vi "CorrFactor.vi"() -> ()   [LabVIEW 2018, in "Visualization.lvlib" / "VisualizeAnalysis.lvclass"]
uses:
  VisualizeAnalysis.lvclass
  VisualizeBase/VisualizeBase_class/SubVIs/VisualizationOptions.ctl
  <vilib>/Utility/miscctls.llb/LVRectTypeDef.ctl
  VisualizeBase/VisualizeBase_class/Requests/VisUserEventType.ctl
  <vilib>/event_ctls.llb/usereventprio.ctl
  <extravilib>/ChannelInstances/Tag-bool/Write With Abort.vi
  <extravilib>/ChannelInstances/Tag-bool/Read With Abort.vi
  <extravilib>/ChannelInstances/Tag-bool/Instantiate.vi
  <extravilib>/ChannelInstances/Tag-bool/EndpointRead.vi
  <vilib>/Utility/error.llb/Error Cluster From Error Code.vi
  <extravilib>/ChannelInstances/Tag-bool/Endpoint.vi
  <vilib>/ErrorRing/Error Ring.xnode
  VisualizeBase/VisualizeBase_class/VisualizeBase.lvclass
  Analysis/AnalysisModule/AnalysisModule.lvlib
  <userlib>/NIST/NISTErrorLib/NISTErrorLib.lvlib
  StatusAndLog/VisualizeStatus.lvclass
  <extravilib>/ChannelInstances/Tag-bool.lvlib
panel:
  in  "Log Data":bool=TRUE
  in  "btnReset":bool
  out "ROCOF":cluster{"Freq":dbl, "Freq":dbl}[](graph)
  out "Freq":cluster{"Freq":dbl, "Freq":dbl}[](graph)
  in  "PluginName":string="Sensor.RoomAlert1"
  in  "btnClearTest":bool
  in  "btnPause":bool
  in  "btnOpen":bool
  in  "INIFilePath":path
  out "VisualizationProperties":T1={"PauseAtStartup"=TRUE, "LogData"=FALSE, "LaunchInSubPanel"=TRUE, "FPMonitor"=0, "FPWindowBounds"={"Left"=0, "Top"=0, "Right"=0, "Bottom"=0}, "MonitorBounds"={"Left"=0, "Top"=0, "Right"=0, "Bottom"=0}}
  in  "ModuleID":i32
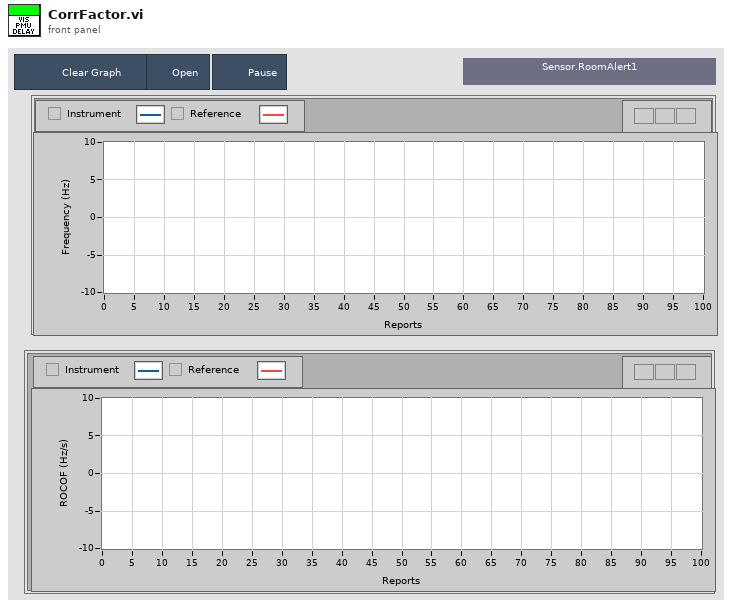
[diagram p1: front panel]
types:
  T1 = typedef "Visualization.lvlib/VisualizeBase.lvclass/VisualizationOptions.ctl" = cluster{"PauseAtStartup":bool, "LogData":bool, "LaunchInSubPanel":bool, "FPMonitor":u16, "FPWindowBounds":T2, "MonitorBounds":cluster{"Left":i16, "Top":i16, "Right":i16, "Bottom":i16}}
  T2 = typedef "LVRectTypeDef.ctl" = cluster{"Left":i16, "Top":i16, "Right":i16, "Bottom":i16}
  T3 = typedef "Visualization.lvlib/VisualizeBase.lvclass/VisRequestEvents.ctl" = cluster{"StopRequest":refnum<user-event>, "ResetRequest":refnum<user-event>, "FP Pop In or Out":refnum<user-event>}
  T4 = typedef "AnalysisModule.lvlib/clBroadcastEvents.ctl" = cluster{"DidInit":refnum<user-event>, "StatusUpdate":refnum<user-event>, "ErrorReport":refnum<user-event>, "DidStop":refnum<user-event>, "PathToINI":refnum<user-event>, "Config":refnum<user-event>, "ResultReport":refnum<user-event>, "FunctionClass":refnum<user-event>, "State":refnum<user-event>, "FunctionParams":refnum<user-event>, "Duration":refnum<user-event>}
  T5 = typedef "usereventprio.ctl" = enum32{"high priority", "normal priority"}
  T6 = typedef "Visualization.lvlib/VisualizeBase.lvclass/VisUserEventType.ctl" = cluster{"BusIndex":i8, "Data":variant}
  T7 = typedef "Tag-bool.lvlib/))Channel.ctl" = refnum<queue>
  T8 = typedef "sizeaction.ctl" = enum32{"Minimized", "Maximized", "Resized"}
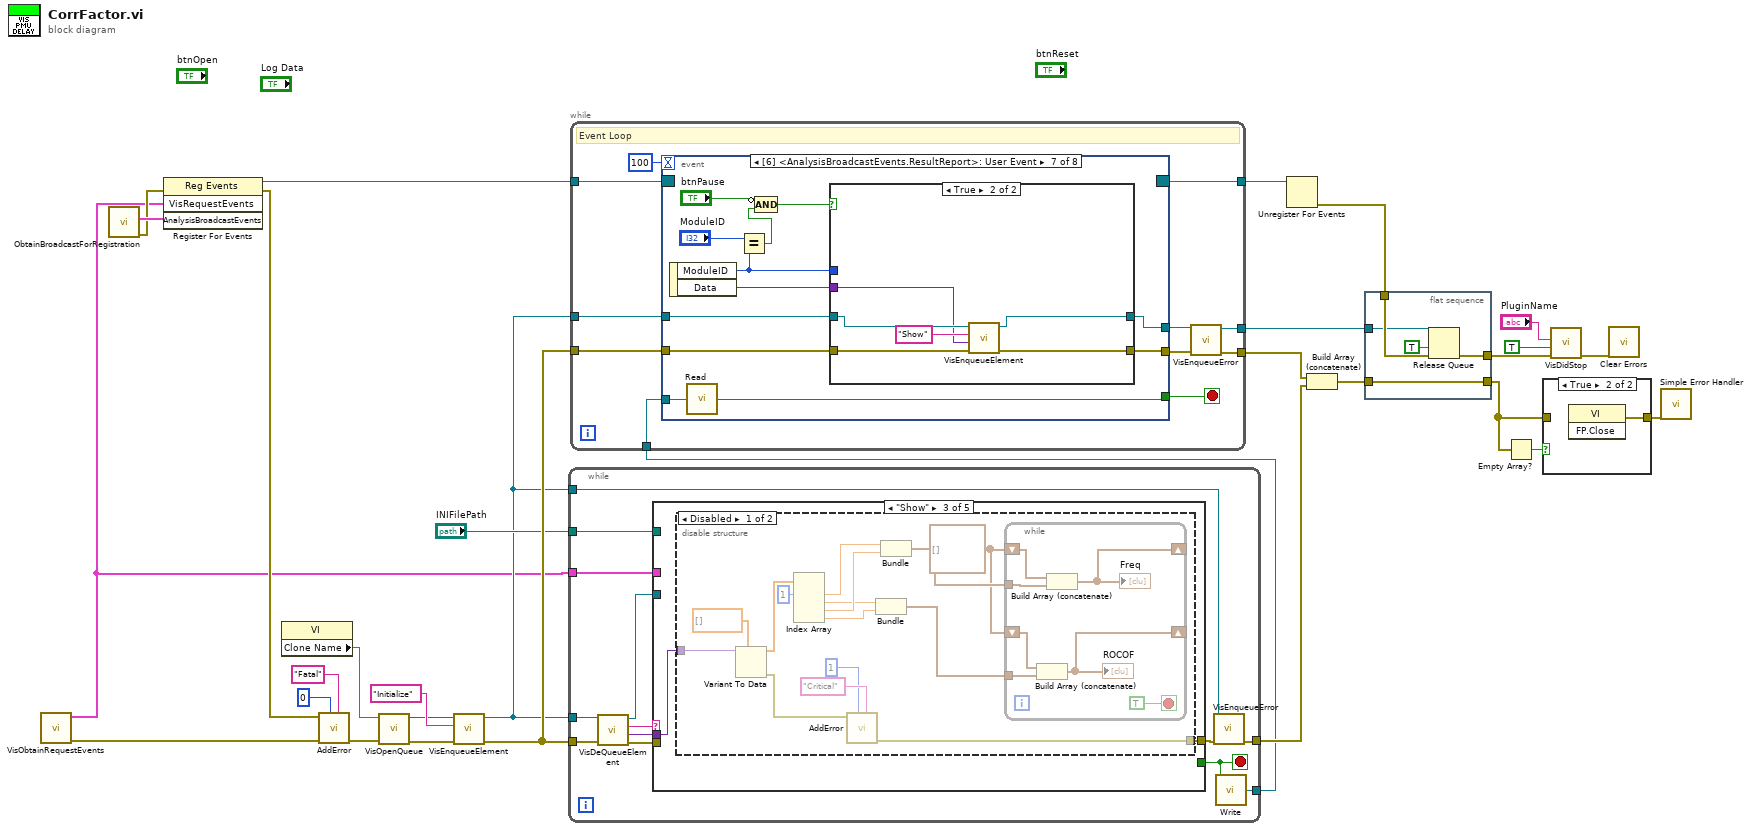
[diagram p0: block diagram]
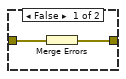
[diagram p2: hidden frame]
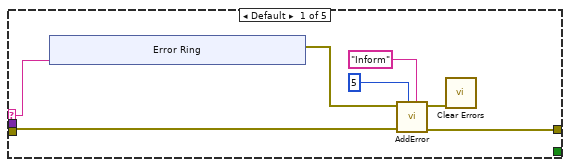
[diagram p3: hidden frame]
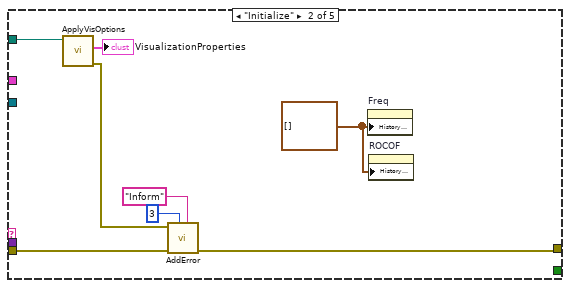
[diagram p4: hidden frame]
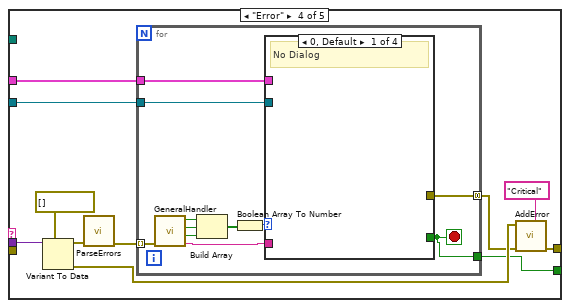
[diagram p6: hidden frame]
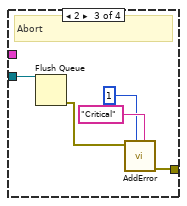
[diagram p8: hidden frame]
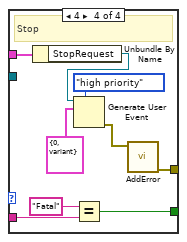
[diagram p9: hidden frame]
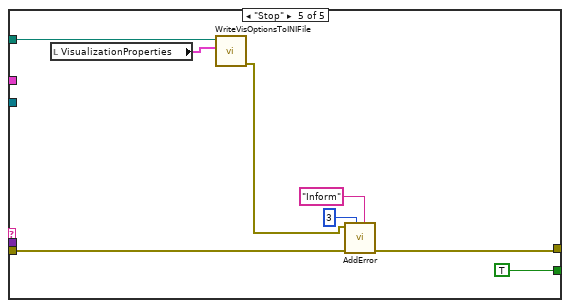
[diagram p10: hidden frame]
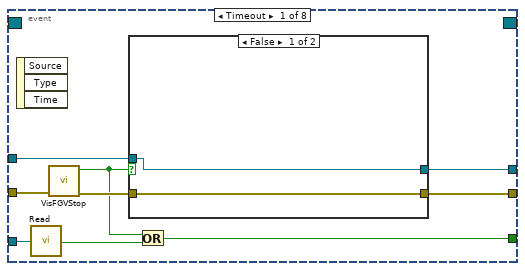
[diagram p11: hidden frame]
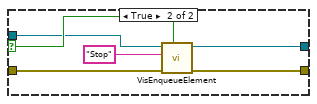
[diagram p12: hidden frame]
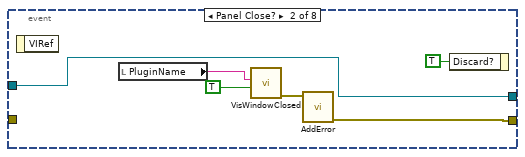
[diagram p13: hidden frame]
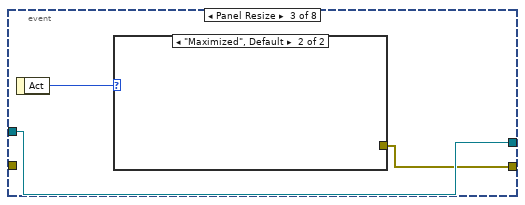
[diagram p14: hidden frame]
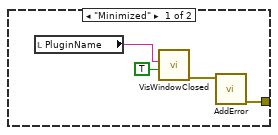
[diagram p15: hidden frame]
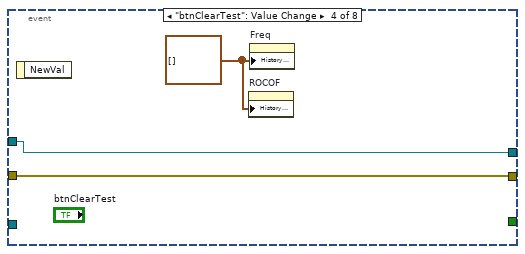
[diagram p16: hidden frame]
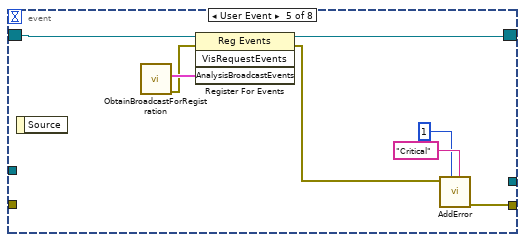
[diagram p17: hidden frame]
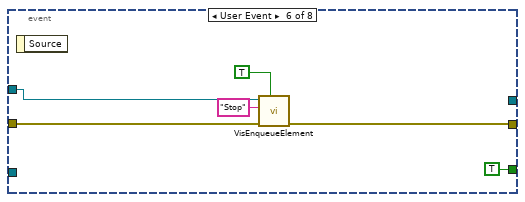
[diagram p18: hidden frame]
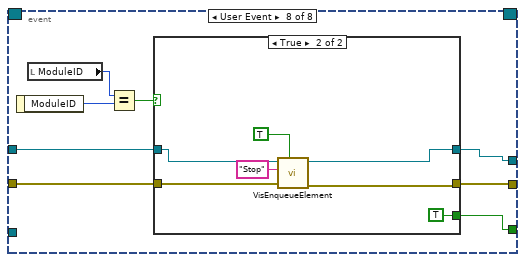
[diagram p20: hidden frame]
diagram:
  n1 = call "VisObtainRequestEvents.vi"() -> ("Error"=w29:errorcluster[], "VisRequestEvents"=w8:T3)  [unwired: 10 in]
  n2 = call "ObtainBroadcastForRegistration.vi"() -> ("error out"=w28:errorcluster, "AnalysisBroadcastEvents"=w30:T4)  [unwired: 10 in]
  n3 = register-events(error in=w28, w8, w30) -> (reference out=w20:refnum<event-registration>, error out=w27:errorcluster)  [unwired: 1 in]
  n4 = property class="VI"() -> ("Clone Name"=w22:string)  [unwired: 2 in, 2 out]
  n5 = call <userlib>:"AddError.vi"("Severity"="Fatal", "Priority"=u8 0, "ErrorArray In"=w29, "error in (no error)"=w27) -> ("ErrorArray Out"=w24:errorcluster[])  [unwired: 6 in, 1 out]
  n6 = call "VisOpenQueue.vi"("Error Array In"=w24, "QueueName"=w22) -> ("Error Array Out"=w23:errorcluster[], "queue out"=w19:refnum<queue>)  [unwired: 8 in]
  n7 = call "VisEnqueueElement.vi"("Error Array In"=w23, "Message"="Initialize", "queue in"=w19) -> ("Error Array Out"=w17:errorcluster[], "queue out"=w9:refnum<queue>)  [unwired: 7 in]
  n8 = while {
    tunnel: w17 -> [w43]
    tunnel: w9 -> [w42]
    tunnel: "INIFilePath" -> [w38]
    tunnel: [w34] -> w12
    tunnel: [w36] -> w10
    tunnel: w9 -> [w33]
    tunnel: w8 -> [w32]
    stop <- w37 stop-if-true
    n9 = call "VisDeQueueElement.vi"("Error Array In"=w43, "Queue In"=w42) -> ("Error Array Out"=w41:errorcluster[], "Data"=w40:variant, "Message"=w39:string, "Queue Out"=w31:refnum<queue>)  [unwired: 6 in]
    n10 = case shown="\"Show\"" w39 {
      selector: w39 -> [w44 _ _ _ _]
      tunnel: w41 -> [w46 w63 _ _ w131]
      tunnel: w40 -> [_ _ w67 w100 _]
      tunnel: w38 -> [_ w65 _ _ w133]
      tunnel: [w45 w59 w66 w95 w127] -> w35
      tunnel: [_ _ _ w92 TRUE] -> w37
      tunnel: w32 -> [_ _ _ w96 _]
      tunnel: w31 -> [_ _ _ w90 _]
      frame Default {
        n11 = xnode "Error Ring"("parameter 0"=w44) -> ("error out"=w50:errorcluster)
        n12 = call <userlib>:"AddError.vi"("Severity"="Inform" ("String"), "Priority"=u8 5, "ErrorArray In"=w46, "error in (no error)"=w50) -> ("ErrorArray Out"=w45:errorcluster[], "error out"=w49:errorcluster)  [unwired: 6 in]
        n13 = call <vilib>:"Clear Errors.vi"("error in (no error)"=w49) -> ()  [unwired: 5 in, 2 out]
      }
      frame "Initialize" {
        w58 = cluster{"Freq":dbl, "Freq":dbl}[] [] ("History Data")
        n14 = call "ApplyVisOptions.vi"("INIFilePath"=w65) -> ("error out"=w62:errorcluster, "VisualizationProperties"=→"VisualizationProperties":T1)  [unwired: 9 in]
        n15 = call <userlib>:"AddError.vi"("Severity"="Inform", "Priority"=u8 3, "ErrorArray In"=w63, "error in (no error)"=w62) -> ("ErrorArray Out"=w59:errorcluster[])  [unwired: 6 in, 1 out]
        n16 = property on="Freq" class="WFChart (strict)"("History Data"=w58) -> ()  [unwired: 2 in, 2 out]
        n17 = property on="ROCOF" class="WFChart (strict)"("History Data"=w58) -> ()  [unwired: 2 in, 2 out]
      }
      frame "Show" {
        n18 = disable-structure shown="Disabled" {
          disable-tunnel: w67 -> [w82 _]
          disable-tunnel: [w80 _] -> w66
          frame Disabled {
            w68 = cluster{"Freq":dbl, "Freq":dbl}[] []
            n19 = Variant To Data(type=dbl[] [], Variant=w82) -> (data=w76:dbl[], error out=w79:errorcluster)  [unwired: 1 in]
            n20 = Index Array(array=w76, index #1=1 ("index")) -> (element #1=w74:dbl, element #2=w72:dbl, element #3=w73:dbl, element #4=w71:dbl)  [unwired: 3 in]
            n21 = call <userlib>:"AddError.vi"("Severity"="Critical", "Priority"=u8 1, "error in (no error)"=w79) -> ("ErrorArray Out"=w80:errorcluster[])  [unwired: 7 in, 1 out]
            n22 = Bundle("Freq"=w72, "Freq"=w71) -> (w69:cluster{"Freq":dbl, "Freq":dbl})  [unwired: 1 in]
            n23 = Bundle("Freq"=w74, "Freq"=w73) -> (w70:cluster{"Freq":dbl, "Freq":dbl})  [unwired: 1 in]
            n24 = while {
              tunnel: w70 -> [w89]
              shift-right: [w87] -> _
              shift-left: w68 -> [w88]
              tunnel: w69 -> [w86]
              shift-right: [w85] -> _
              shift-left: w68 -> [w84]
              stop <- TRUE stop-if-true
              n25 = Build Array (concatenate)(w84, w86) -> (w85:cluster{"Freq":dbl, "Freq":dbl}[])
              "ROCOF" <- w85
              n26 = Build Array (concatenate)(w88, w89) -> (w87:cluster{"Freq":dbl, "Freq":dbl}[])
              "Freq" <- w87
            }
          }
          frame Enabled {
          }
        }
      }
      frame "Error" {
        n27 = Variant To Data(type=errorcluster[] [], Variant=w100) -> (data=w98:errorcluster[], error out=w94:errorcluster)  [unwired: 1 in]
        n28 = call <userlib>:"ParseErrors.vi"("ErrorArray"=w98) -> ("ErrorArray"=w97:errorcluster[])  [unwired: 8 in, 2 out]
        n29 = for {
          tunnel: w97 -> [w111] mode=indexing
          tunnel: w96 -> [w106]
          tunnel: [w103] -> w92
          tunnel: [w102] -> w91 mode=concatenating
          tunnel: w90 -> [w101]
          stop <- w103 stop-if-true
          n30 = call <userlib>:"GeneralHandler.vi"("error in (no error)"=w111) -> ("Severity"=w104:string, "Stop"=w110:bool, "Abort"=w109:bool, "Continue"=w108:bool)  [unwired: 6 in, 1 out]
          n31 = Build Array(w108, w109, w110) -> (w107:bool[])
          n32 = Boolean Array To Number(Boolean array=w107) -> (number=w105:u32)
          n33 = case shown="0, Default" w105 {
            tunnel: w106 -> [_ _ _ w125]
            tunnel: w104 -> [_ _ _ w121]
            tunnel: [_ _ _ w119] -> w103
            tunnel: [_ _ w115 w117] -> w102
            tunnel: w101 -> [_ _ w116 _]
            frame 0, Default {
              # "No Dialog"
            }
            frame 1 {
              # "Continue"
            }
            frame 2 {
              # "Abort"
              n34 = Flush Queue(queue=w116) -> (error out=w114:errorcluster)  [unwired: 1 in, 2 out]
              n35 = call <userlib>:"AddError.vi"("Severity"="Critical", "Priority"=u8 1, "error in (no error)"=w114) -> ("ErrorArray Out"=w115:errorcluster[])  [unwired: 7 in, 1 out]
            }
            frame 4 {
              # "Stop"
              n36 = Unbundle By Name(w125) -> ("StopRequest"=w123:refnum<user-event>)
              n37 = Generate User Event(priority (normal)=usereventprio."high priority", user event=w123, event data cluster=T6 {"BusIndex"=0, "Data"=variant} ("event data")) -> (error out=w118:errorcluster)  [unwired: 1 in, 1 out]
              n38 = Equal?(x="Fatal", y=w121) -> (x = y?=w119:bool)
              n39 = call <userlib>:"AddError.vi"("error in (no error)"=w118) -> ("ErrorArray Out"=w117:errorcluster[])  [unwired: 9 in, 1 out]
            }
          }
        }
        n40 = call <userlib>:"AddError.vi"("Severity"="Critical", "ErrorArray In"=w91, "error in (no error)"=w94) -> ("ErrorArray Out"=w95:errorcluster[])  [unwired: 7 in, 1 out]
      }
      frame "Stop" {
        n41 = local read "VisualizationProperties"() -> (w132:T1)
        n42 = call "WriteVisOptionsToINIFile.vi"("Visualization Options"=w132, "INIFilePath"=w133) -> ("error out"=w128:errorcluster)  [unwired: 8 in, 1 out]
        n43 = call <userlib>:"AddError.vi"("Severity"="Inform", "Priority"=u8 3, "ErrorArray In"=w131, "error in (no error)"=w128) -> ("ErrorArray Out"=w127:errorcluster[])  [unwired: 6 in, 1 out]
      }
    }
    n44 = call "VisEnqueueError.vi"("Error Array In"=w35, "Queue in"=w33) -> ("Error Array Out"=w34:errorcluster[])  [unwired: 8 in, 1 out]
    n45 = call <extravilib>:"Write.vi"("element"=w37) -> ("channel"=w36:T7)  [unwired: 1 out]
  }
  n46 = while {
    tunnel: w20 -> [w143]
    tunnel: w17 -> [w142]
    tunnel: w9 -> [w141]
    tunnel: [w137] -> w13
    tunnel: [w136] -> w15
    tunnel: [w135] -> w18
    tunnel: w10 -> [w134]
    stop <- w138 stop-if-true
    # "Event Loop"
    n47 = event shown="[6] <AnalysisBroadcastEvents.ResultReport>: User Event" {
      selector: w143 -> [_ _ _ _ w185 _ _ _]
      dyn-events: [_ _ _ _ w182 _ _ _] -> w135
      timeout: 100 -> [_ _ _ _ _ _ _ _]
      tunnel: w142 -> [w153 _ _ w176 _ w191 w193 w215]
      tunnel: w141 -> [w151 w162 w170 w177 _ w187 w195 w216]
      tunnel: [w150 w162 w170 w177 _ _ w194 w214] -> w140
      tunnel: [w149 w165 w168 w176 w181 w188 w192 w213] -> w139
      tunnel: [w147 _ _ _ _ TRUE w202 w212] -> w138
      tunnel: w134 -> [w146 _ _ _ _ _ w203 _]
      event Timeout {
        n48 = event-data() -> ()  [unwired: 1 in, 3 out]
        n49 = call <extravilib>:"Read.vi"("channel"=w146) -> ("element"=w145:bool)  [unwired: 1 in, 1 out]
        n50 = call "VisFGVStop.vi"("Error In"=w153) -> ("Error Out"=w152:errorcluster[], "Value"=w148:bool)  [unwired: 9 in]
        n51 = case shown="False" w148 {
          selector: w148 -> [_ w159]
          tunnel: w152 -> [w155 w161]
          tunnel: w151 -> [w154 w158]
          tunnel: [w154 w157] -> w150
          tunnel: [w155 w156] -> w149
          frame False {
          }
          frame True {
            n52 = call "VisEnqueueElement.vi"("Priority? (F)"=w159, "Error Array In"=w161, "Message"="Stop", "queue in"=w158) -> ("Error Array Out"=w156:errorcluster[], "queue out"=w157:refnum<queue>)  [unwired: 6 in]
          }
        }
        n53 = Or(x=w148, y=w145) -> (x .or. y?=w147:bool)
      }
      event Panel Close? {
        n54 = event-data() -> ()  [unwired: 1 in, 1 out]
        n55 = local read "PluginName"() -> (w167:string)
        n56 = call "VisWindowClosed.vi"("Window Closed?"=TRUE, "Module Name"=w167) -> ("error out"=w164:errorcluster)  [unwired: 9 in]
        n57 = call <userlib>:"AddError.vi"("error in (no error)"=w164) -> ("ErrorArray Out"=w165:errorcluster[])  [unwired: 9 in, 1 out]
        n58 = event-data("Discard?"=TRUE) -> ()  [unwired: 1 in, 1 out]
      }
      event Panel Resize {
        n59 = event-data() -> ("Act"=w169:T8)  [unwired: 1 in]
        n60 = case shown="\"Maximized\", Default" w169 {
          tunnel: [w171 _] -> w168
          frame "Minimized" {
            n61 = local read "PluginName"() -> (w174:string)
            n62 = call "VisWindowClosed.vi"("Window Closed?"=TRUE, "Module Name"=w174) -> ("error out"=w172:errorcluster)  [unwired: 9 in]
            n63 = call <userlib>:"AddError.vi"("error in (no error)"=w172) -> ("ErrorArray Out"=w171:errorcluster[])  [unwired: 9 in, 1 out]
          }
          frame "Maximized", Default {
          }
        }
      }
      event "btnClearTest": Value Change {
        w175 = cluster{"Freq":dbl, "Freq":dbl}[] [] ("History Data")
        n64 = event-data() -> ()  [unwired: 1 in, 1 out]
        n65 = property on="ROCOF" class="WFChart (strict)"("History Data"=w175) -> ()  [unwired: 2 in, 2 out]
        n66 = property on="Freq" class="WFChart (strict)"("History Data"=w175) -> ()  [unwired: 2 in, 2 out]
      }
      event User Event {
        n67 = event-data() -> ()  [unwired: 1 in, 1 out]
        n68 = call "ObtainBroadcastForRegistration.vi"() -> ("error out"=w183:errorcluster, "AnalysisBroadcastEvents"=w184:T4)  [unwired: 10 in]
        n69 = register-events(reference=w185, error in=w183, w184) -> (reference out=w182:refnum<event-registration>, error out=w180:errorcluster)  [unwired: 1 in]
        n70 = call <userlib>:"AddError.vi"("Severity"="Critical", "Priority"=u8 1, "error in (no error)"=w180) -> ("ErrorArray Out"=w181:errorcluster[])  [unwired: 7 in, 1 out]
      }
      event User Event {
        n71 = event-data() -> ()  [unwired: 1 in, 1 out]
        n72 = call "VisEnqueueElement.vi"("Priority? (F)"=TRUE, "Error Array In"=w191, "Message"="Stop", "queue in"=w187) -> ("Error Array Out"=w188:errorcluster[])  [unwired: 6 in, 1 out]
      }
      event User Event {
        n73 = event-data() -> ("ModuleID"=w200:i32, "Data"=w201:variant)  [unwired: 1 in]
        n74 = call <extravilib>:"Read.vi"("channel"=w203) -> ("element"=w202:bool)  [unwired: 1 in, 1 out]
        n75 = Equal?(x="ModuleID", y=w200) -> (x = y?=w197:bool)
        n76 = Compound Arithmetic op=AND(invert "btnPause", w197) -> (w196:bool)
        n77 = case shown="True" w196 {
          tunnel: w200 -> [_ _]
          tunnel: w201 -> [_ w206]
          tunnel: [w205 w208] -> w194
          tunnel: w195 -> [w205 w210]
          tunnel: w193 -> [w204 w211]
          tunnel: [w204 w209] -> w192
          frame False {
          }
          frame True {
            n78 = call "VisEnqueueElement.vi"("Error Array In"=w211, "Data"=w206, "Message"="Show", "queue in"=w210) -> ("Error Array Out"=w209:errorcluster[], "queue out"=w208:refnum<queue>)  [unwired: 6 in]
          }
        }
      }
      event User Event {
        n79 = event-data() -> ("ModuleID"=w219:i32)  [unwired: 1 in]
        n80 = local read "ModuleID"() -> (w218:i32)
        n81 = Equal?(x=w218, y=w219) -> (x = y?=w217:bool)
        n82 = case shown="True" w217 {
          tunnel: w216 -> [w222 w228]
          tunnel: w215 -> [w221 w229]
          tunnel: [w222 w226] -> w214
          tunnel: [w221 w227] -> w213
          tunnel: [FALSE TRUE] -> w212
          frame False {
          }
          frame True {
            n83 = call "VisEnqueueElement.vi"("Priority? (F)"=TRUE, "Error Array In"=w229, "Message"="Stop", "queue in"=w228) -> ("Error Array Out"=w227:errorcluster[], "queue out"=w226:refnum<queue>)  [unwired: 6 in]
          }
        }
      }
    }
    n84 = call "VisEnqueueError.vi"("Error Array In"=w139, "Queue in"=w140) -> ("Error Array Out"=w137:errorcluster[], "Queue out"=w136:refnum<queue>)  [unwired: 8 in]
  }
  n85 = Unregister For Events(event registration refnum=w18) -> (error out=w16:errorcluster)  [unwired: 1 in]
  n86 = Build Array (concatenate)(w13, w12) -> (w11:errorcluster[])
  n87 = flat-sequence {
    tunnel: w16 -> [w234]
    tunnel: w15 -> [w232]
    tunnel: [w231] -> w2
    tunnel: w11 -> [w231]
    tunnel: [w230] -> w7
    frame #0 {
      n88 = Release Queue(queue=w232, force destroy? (F)=TRUE, error in (no error)=w234) -> (error out=w230:errorcluster)  [unwired: 2 out]
    }
  }
  n89 = Empty Array?(array=w2) -> (empty?=w4:bool)
  n90 = case shown="True" w4 {
    tunnel: w2 -> [w236 _]
    tunnel: [w235 w237] -> w1
    frame False {
      n91 = Merge Errors(w236) -> (w235:errorcluster)
    }
    frame True {
      n92 = invoke class="VI" method="FP.Close"() -> (error out=w237:errorcluster)  [unwired: 3 in, 2 out]
    }
  }
  n93 = call "VisDidStop.vi"("error in (no error)"=w7, "DidStop?"=TRUE, "Module Name"="PluginName") -> ("error out"=w3:errorcluster)  [unwired: 8 in]
  n94 = call <vilib>:"Clear Errors.vi"("error in (no error)"=w3) -> ()  [unwired: 5 in, 2 out]
  n95 = call <vilib>:"Simple Error Handler.vi"("error in (no error)"=w1) -> ()  [unwired: 4 in, 5 out]
